vi "FreeMemInfo.vi"() -> (1 "PhysicalSpace":dbl format="%.2f", 2 "PhysicalFreeSpace":dbl format="%.2f")   [LabVIEW 2015]
uses:
  lv64_eventdriven/board.vis/ESLSCDLL.dll
panel:
  # "MB"
  # "MB"
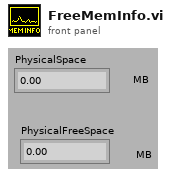
[diagram p1: front panel]
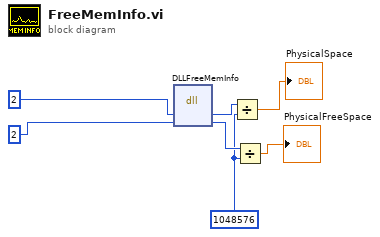
[diagram p0: block diagram]
diagram:
  w3 = 1048576
  n1 = dll-call lib="C:/ENTW/PCIE/64bit/lv64/lv64_eventdriven/board.vis/ESLSCDLL.dll" fn="DLLFreeMemInfo"("memory_all"=u32 2, "memory_free"=u32 2) -> ("memory_all"=w5:u64, "memory_free"=w4:u64)  [unwired: 4 in, 2 out]
  n2 = Divide(x=w5, y=w3) -> (x/y=→"PhysicalSpace":dbl)
  n3 = Divide(x=w4, y=w3) -> (x/y=→"PhysicalFreeSpace":dbl)
